vi "RT Loop - Acquisition and Logging.vi"(8 "error in (no error)":errorcluster, 9 "Acquisition and Logging Configuration":T1={"Data Rate"=1, "Samples per Read"=0, "Number of Reads to Save"=0, "Data File Name"="", "TDMS Properties"=[], "Number of Channels"=4, "Channel Scale Array"=[0.0, 0.0, 0.0, 0.0], "Channel Names"=[], "Trigger - RMS Value"=0.0, "Trigger - Channel"=0, "Trigger - Time (Minute)"=0} {"Data Rate" items=["51.200 kS/s (NI 9234)"=1, "25.600 kS/s (NI 9234)"=2, "17.067 kS/s (NI 9234)"=3, "12.800 kS/s (NI 9234)"=4, "10.240 kS/s (NI 9234)"=5, "8.533 kS/s (NI 9234)"=6, "7.314 kS/s (NI 9234)"=7, "6.400 kS/s (NI 9234)"=8, "5.689 kS/s (NI 9234)"=9, "5.120 kS/s (NI 9234)"=10, "4.654 kS/s (NI 9234)"=11, "4.267 kS/s (NI 9234)"=12, "3.938 kS/s (NI 9234)"=13, "3.657 kS/s (NI 9234)"=14, "3.413 kS/s (NI 9234)"=15, "3.200 kS/s (NI 9234)"=16, "3.012 kS/s (NI 9234)"=17, "2.845 kS/s (NI 9234)"=18, "2.695 kS/s (NI 9234)"=19, "2.560 kS/s (NI 9234)"=20, "2.438 kS/s (NI 9234)"=21, "2.328 kS/s (NI 9234)"=22, "2.226 kS/s (NI 9234)"=23, "2.133 kS/s (NI 9234)"=24, "2.048 kS/s (NI 9234)"=25, "1.969 kS/s (NI 9234)"=26, "1.896 kS/s (NI 9234)"=27, "1.829 kS/s (NI 9234)"=28, "1.765 kS/s (NI 9234)"=29, "1.707 kS/s (NI 9234)"=30, "1.652 kS/s (NI 9234)"=31]}, 10 "Acquisition and Logging Queue":refnum<queue>, 11 "Message Queue":refnum<queue>) -> ()   [LabVIEW 2020]
uses:
  support/Message Queue/Message Cluster.ctl
  controls/Acquisition and Logging Configuration.ctl
  <vilib>/LabVIEW Targets/FPGA/cRIO/shared/nicrio_ModuleControls/nicrio_cRIO-9234_DataRatesRing2.ctl
  controls/TDMS Properties.ctl
  controls/FPGA VI Reference.ctl
  Globals/Global - Configuration Options.vi
  Globals/Global - Monitoring Variables.vi
  <vilib>/rvi/errors/niLvFpgaAdjustHostInterfaceError.vi
  <vilib>/rvi/interface/nirviReadWriteControl/nirviReadWriteControl.xnode
  FPGA Bitfiles/forthexerciseemc_FPGATarget2_FPGAMain_d5JOh9LSVOQ.lvbitx
  support/Message Queue/Message Queue.lvlib
  NiFpgaLv.dll
panel:
  in  "Unbalanced Fan Speed 2":fxp<+/-,20,5>
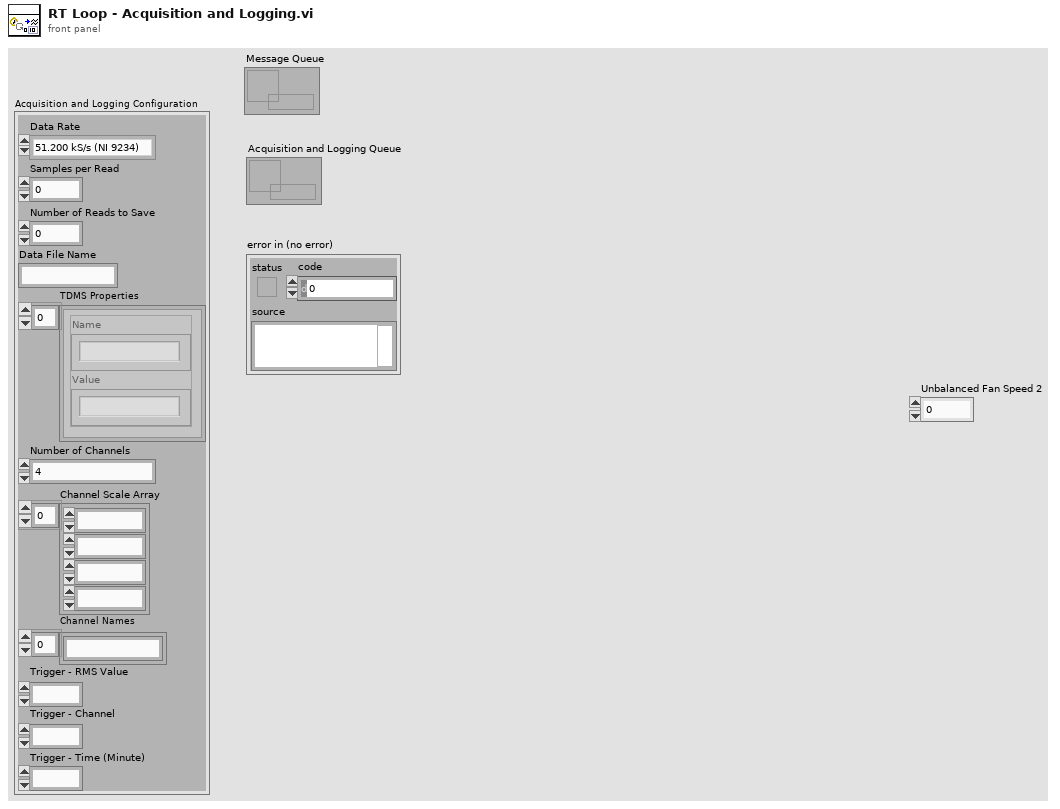
[diagram p1: front panel]
types:
  T1 = typedef "Acquisition and Logging Configuration.ctl" = cluster{"Data Rate":T2, "Samples per Read":i32, "Number of Reads to Save":i32, "Data File Name":string, "TDMS Properties":T3[], "Number of Channels":i32, "Channel Scale Array":fxp<+,24,12>[], "Channel Names":string[], "Trigger - RMS Value":dbl, "Trigger - Channel":i32, "Trigger - Time (Minute)":i32}
  T2 = typedef "nicrio_cRIO-9234_DataRatesRing2.ctl" = u8
  T3 = typedef "TDMS Properties.ctl" = cluster{"Name":string, "Value":string}
  T4 = typedef "FPGA VI Reference.ctl" = refnum<k20>
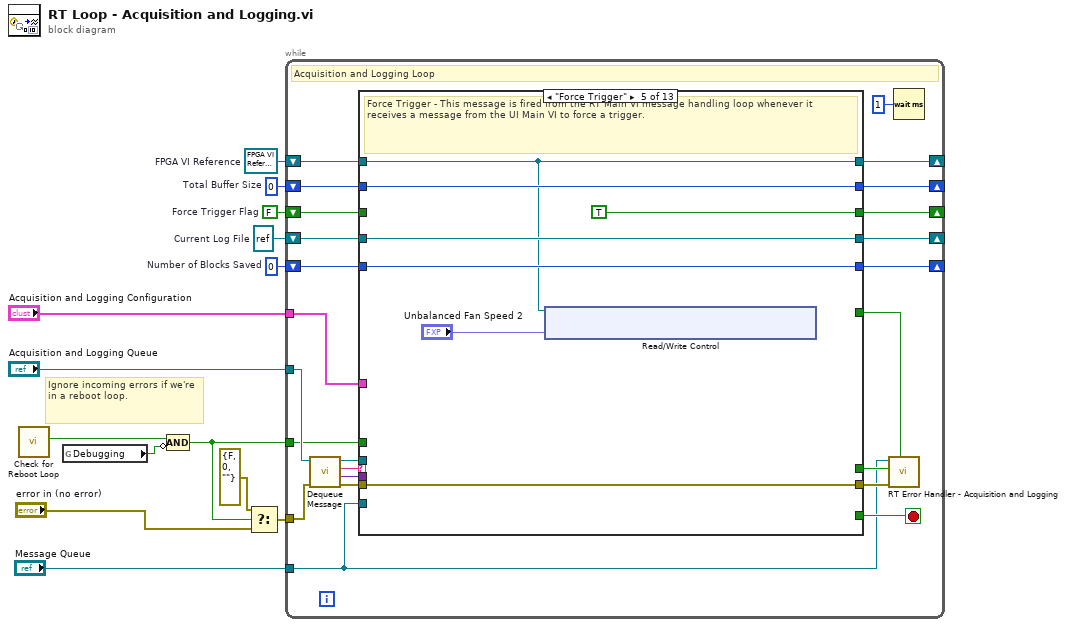
[diagram p0: block diagram]
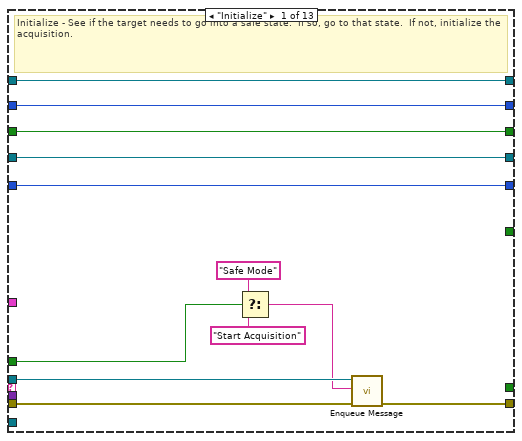
[diagram p2: hidden frame]
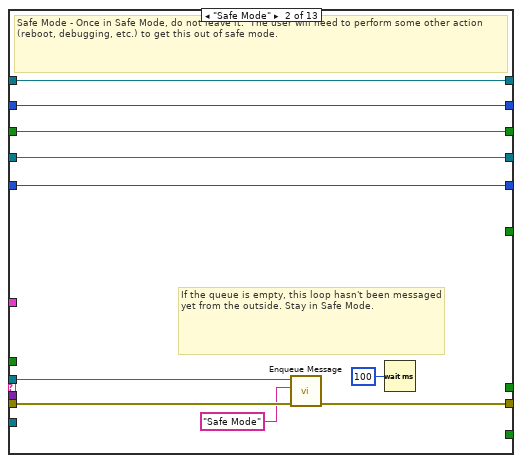
[diagram p3: hidden frame]
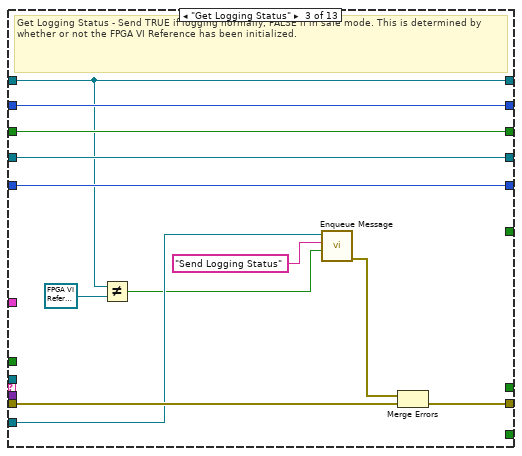
[diagram p4: hidden frame]
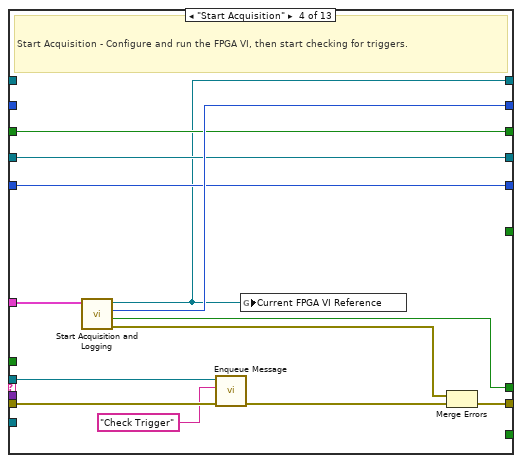
[diagram p5: hidden frame]
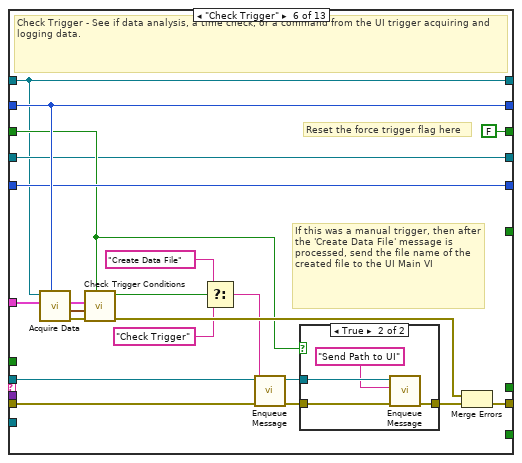
[diagram p6: hidden frame]
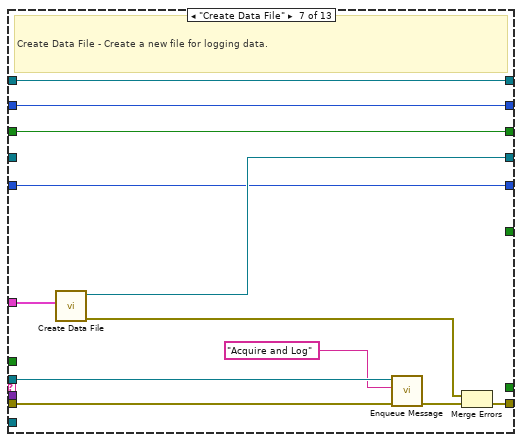
[diagram p8: hidden frame]
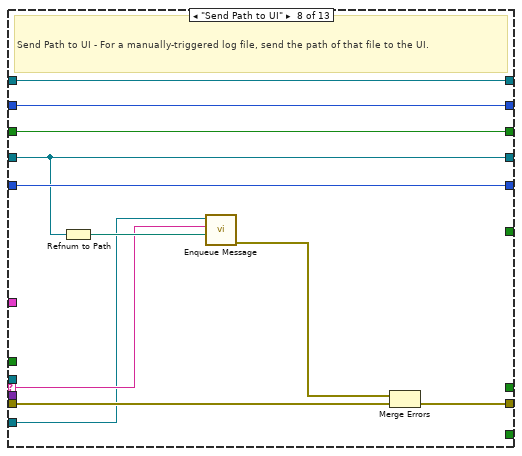
[diagram p9: hidden frame]
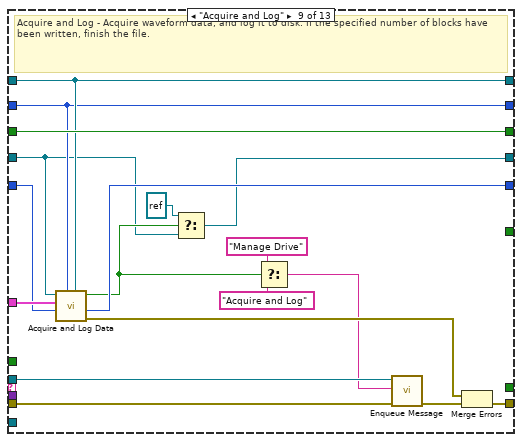
[diagram p10: hidden frame]
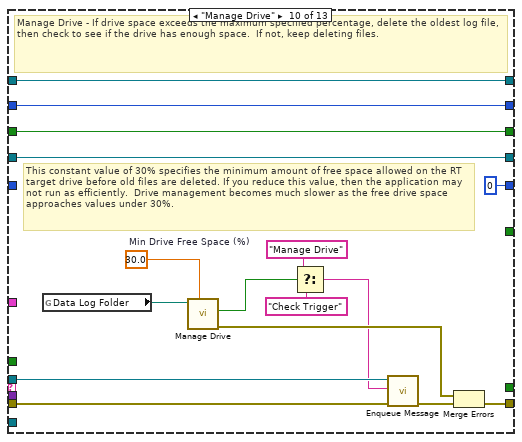
[diagram p11: hidden frame]
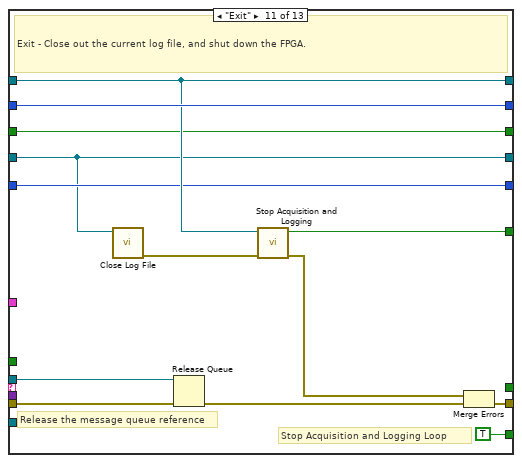
[diagram p12: hidden frame]
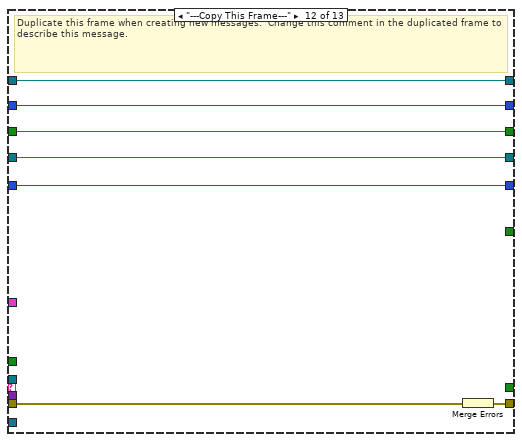
[diagram p13: hidden frame]
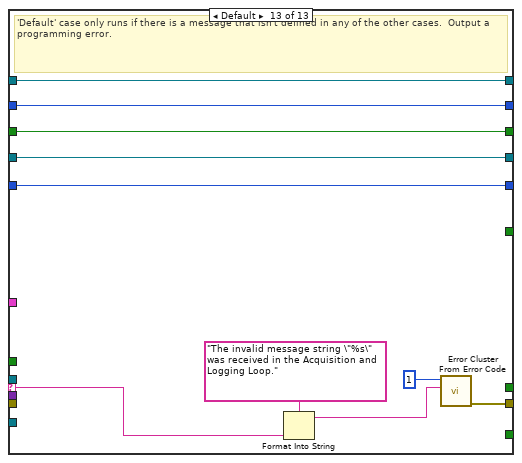
[diagram p14: hidden frame]
diagram:
  w7 = 0  # Number of Blocks Saved
  w8 = refnum<k34> refnum  # Current Log File
  w9 = FALSE  # Force Trigger Flag
  w11 = 0  # Total Buffer Size
  w12 = T4 refnum  # FPGA VI Reference
  # "Ignore incoming errors if we're in a reboot loop."
  n1 = call "Check for Reboot Loop.vi"() -> ("Start in Safe Mode?"=w3:bool)  [unwired: 10 in, 1 out]
  n2 = global read "Global - Configuration Options.vi" "Debugging"() -> (w2:bool)
  n3 = Compound Arithmetic op=AND(w3, invert w2) -> (w1:bool)
  n4 = Select(t=errorcluster {"status"=FALSE, "code"=0, "source"=""}, s=w1, f="error in (no error)") -> (s? t:f=w5:errorcluster)
  n5 = while {
    tunnel: "Acquisition and Logging Queue" -> [w34]
    tunnel: "Message Queue" -> [w18]
    shift-right: [w29] -> _
    shift-left: w12 -> [w31]
    shift-right: [w28] -> _
    shift-left: w11 -> [w30]
    tunnel: "Acquisition and Logging Configuration" -> [w27]
    shift-right: [w23] -> _
    shift-left: w9 -> [w24]
    shift-right: [w21] -> _
    shift-left: w8 -> [w22]
    shift-right: [w19] -> _
    shift-left: w7 -> [w20]
    tunnel: w5 -> [w16]
    tunnel: w1 -> [w15]
    stop <- w38 stop-if-true
    # "Acquisition and Logging Loop"
    n6 = call "Dequeue Message.vi"("error in (no error)"=w16, "Message Queue"=w34) -> ("error out"=w37:errorcluster, "Message Data"=w35:variant, "Message"=w36:string, "dup Message Queue"=w32:refnum<queue>)  [unwired: 6 in]
    n7 = case "Message Cases" shown="\"Force Trigger\"" w36 {
      selector: w36 -> [_ _ _ _ _ _ _ w134 _ _ _ _ w204]
      tunnel: w32 -> [w47 w57 _ w78 _ w105 w125 _ w156 w168 w188 _ _]
      tunnel: w37 -> [w48 w58 w72 w85 w92 w113 w129 w141 w159 w175 w184 w195 _]
      tunnel: [w40 w56 w64 w83 w92 w112 w128 w132 w158 w171 w185 w194 w202] -> w33
      tunnel: [_ _ _ _ _ _ _ _ _ _ TRUE _ _] -> w38
      tunnel: w35 -> [_ _ _ _ _ _ _ _ _ _ _ _ _]
      tunnel: w31 -> [w50 w60 w67 _ w86 w93 w130 w140 w149 w174 w182 w193 w200]
      tunnel: w30 -> [w49 w59 w71 _ w91 w110 w127 w139 w148 w173 w183 w192 w199]
      tunnel: [w50 w60 w67 w73 w86 w93 w130 w140 w149 w174 w182 w193 w200] -> w29
      tunnel: [w49 w59 w71 w80 w91 w110 w127 w139 w148 w173 w183 w192 w199] -> w28
      tunnel: w27 -> [_ _ _ w84 _ w111 w122 _ w154 _ _ _ _]
      tunnel: [_ _ _ w81 _ _ _ _ _ _ _ _ _] -> w25
      tunnel: w24 -> [w43 w55 w70 w76 _ w95 w123 w138 w155 w161 w180 w191 w198]
      tunnel: [w43 w55 w70 w76 TRUE ("Force Trigger Flag") FALSE ("Force Trigger Flag") w123 w138 w155 w161 w180 w191 w198] -> w23
      tunnel: w22 -> [w42 w54 w69 w75 w90 w94 _ w136 w144 w172 w177 w190 w197]
      tunnel: [w42 w54 w69 w75 w90 w94 w120 w136 w143 w172 w177 w190 w197] -> w21
      tunnel: w20 -> [w41 w53 w68 w74 w88 w100 w119 w137 w147 _ w179 w189 w196]
      tunnel: [w41 w53 w68 w74 w88 w100 w119 w137 w146 0 ("Number of Blocks Saved") w179 w189 w196] -> w19
      tunnel: w18 -> [_ _ w65 _ _ _ _ w133 _ _ _ _ _]
      tunnel: [_ _ _ _ _ _ _ _ _ _ w176 _ _] -> w17
      tunnel: w15 -> [w39 _ _ _ _ _ _ _ _ _ _ _ _]
      frame "Initialize" {
        # "Initialize - See if the target needs to go into a safe state.  If so, go to that state.  If not, initialize the acquisition."
        n8 = Select(t="Safe Mode", s=w39, f="Start Acquisition") -> (s? t:f=w44:string)
        n9 = call "Enqueue Message.vi"("error in (no error)"=w48, "Message"=w44, "Message Queue"=w47) -> ("error out"=w40:errorcluster)  [unwired: 7 in, 1 out]
      }
      frame "Safe Mode" {
        # "If the queue is empty, this loop hasn't been messaged yet from the outside. Stay in Safe Mode."
        # "Safe Mode - Once in Safe Mode, do not leave it.  The user will need to perform some other action (reboot, debugging, etc.) to get this out of safe mode."
        n10 = call "Enqueue Message.vi"("error in (no error)"=w58, "Message"="Safe Mode", "Message Queue"=w57) -> ("error out"=w56:errorcluster)  [unwired: 7 in, 1 out]
        n11 = Wait (ms)(milliseconds to wait=u32 100) -> ()  [unwired: 1 out]
      }
      frame "Get Logging Status" {
        # "Get Logging Status - Send TRUE if logging normally, FALSE if in safe mode. This is determined by whether or not the FPGA VI Reference has been initialized."
        n12 = Not Equal?(x=w67, y=T4 refnum ("FPGA VI Reference")) -> (x != y?=w62:bool)
        n13 = call "Enqueue Message.vi"("Message Data"=w62, "Message"="Send Logging Status", "Message Queue"=w65) -> ("error out"=w63:errorcluster)  [unwired: 7 in, 1 out]
        n14 = Merge Errors(w63, w72) -> (w64:errorcluster)
      }
      frame "Start Acquisition" {
        # "Start Acquisition - Configure and run the FPGA VI, then start checking for triggers."
        n15 = call "Start Acquisition and Logging.vi"("Acquisition and Logging Configuration"=w84) -> ("error out"=w82:errorcluster, "Wait on IRQ Timeout?"=w81:bool, "Total Buffer Size"=w80:i32, "FPGA VI Reference Out"=w73:T4)  [unwired: 7 in]
        n16 = call "Enqueue Message.vi"("error in (no error)"=w85, "Message"="Check Trigger", "Message Queue"=w78) -> ("error out"=w79:errorcluster)  [unwired: 7 in, 1 out]
        n17 = global write "Global - Monitoring Variables.vi" "Current FPGA VI Reference"(w73) -> ()
        n18 = Merge Errors(w82, w79) -> (w83:errorcluster)
      }
      frame "Force Trigger" {
        # "Force Trigger - This message is fired from the RT Main VI message handling loop whenever it receives a message from the UI Main VI to force a trigger."
        n19 = xnode "Read/Write Control"("FPGA VI Reference In"=w86, "Unbalanced Fan Speed"="Unbalanced Fan Speed 2") -> ()  [unwired: 1 in, 2 out]
      }
      frame "Check Trigger" {
        # "If this was a manual trigger, then after the 'Create Data File' message is processed, send the file name of the created file to the UI Main VI"
        # "Reset the force trigger flag here"
        # "Check Trigger - See if data analysis, a time check, or a command from the UI trigger acquiring and logging data."
        n20 = call "Acquire Data.vi"("Total Buffer Size"=w110, "Acquisition and Logging Configuration"=w111, "FPGA VI Reference"=w93) -> ("error out"=w108:errorcluster, "Waveform Data"=w107:waveform(sgl)[], "dup Acquisition and Logging Configuration"=w106:T1)  [unwired: 6 in]
        n21 = call "Check Trigger Conditions.vi"("Force Trigger?"=w95, "error in (no error)"=w108, "Waveform Data"=w107, "Acquisition and Logging Configuration"=w106) -> ("error out"=w109:errorcluster, "Trigger Condition Met?"=w104:bool)  [unwired: 6 in]
        n22 = Select(t="Create Data File", s=w104, f="Check Trigger") -> (s? t:f=w101:string)
        n23 = call "Enqueue Message.vi"("error in (no error)"=w113, "Message"=w101, "Message Queue"=w105) -> ("error out"=w98:errorcluster, "dup Message Queue"=w96:refnum<queue>)  [unwired: 7 in]
        n24 = case shown="True" w95 {
          tunnel: w98 -> [w114 w117]
          tunnel: [w114 w118] -> w97
          tunnel: w96 -> [_ w116]
          frame False {
          }
          frame True {
            n25 = call "Enqueue Message.vi"("error in (no error)"=w117, "Message"="Send Path to UI", "Message Queue"=w116) -> ("error out"=w118:errorcluster)  [unwired: 7 in, 1 out]
          }
        }
        n26 = Merge Errors(w109, w97) -> (w112:errorcluster)
      }
      frame "Create Data File" {
        # "Create Data File - Create a new file for logging data."
        n27 = call "Create Data File.vi"("Acquisition and Logging Configuration"=w122) -> ("error out"=w121:errorcluster, "TDMS File Reference"=w120:refnum<k34>)  [unwired: 9 in]
        n28 = call "Enqueue Message.vi"("error in (no error)"=w129, "Message"="Acquire and Log", "Message Queue"=w125) -> ("error out"=w126:errorcluster)  [unwired: 7 in, 1 out]
        n29 = Merge Errors(w121, w126) -> (w128:errorcluster)
      }
      frame "Send Path to UI" {
        # "Send Path to UI - For a manually-triggered log file, send the path of that file to the UI."
        n30 = Refnum to Path(1:w136) -> (0:w135:path)
        n31 = call "Enqueue Message.vi"("Message Data"=w135, "Message"=w134, "Message Queue"=w133) -> ("error out"=w131:errorcluster)  [unwired: 7 in, 1 out]
        n32 = Merge Errors(w131, w141) -> (w132:errorcluster)
      }
      frame "Acquire and Log" {
        # "Acquire and Log - Acquire waveform data, and log it to disk. If the specified number of blocks have been written, finish the file."
        n33 = call "Acquire and Log Data.vi"("FPGA VI Reference"=w149, "Total Buffer Size"=w148, "Number of Blocks Saved in"=w147, "Acquisition and Logging Configuration"=w154, "TDMS File Reference"=w144) -> ("error out"=w153:errorcluster, "Number of Blocks Saved out"=w146:i32, "Logging Complete?"=w145:bool)  [unwired: 4 in]
        n34 = Select(t=refnum<k34> refnum, s=w145, f=w144) -> (s? t:f=w143:refnum<k34>)
        n35 = Select(t="Manage Drive", s=w145, f="Acquire and Log") -> (s? t:f=w150:string)
        n36 = call "Enqueue Message.vi"("error in (no error)"=w159, "Message"=w150, "Message Queue"=w156) -> ("error out"=w157:errorcluster)  [unwired: 7 in, 1 out]
        n37 = Merge Errors(w153, w157) -> (w158:errorcluster)
      }
      frame "Manage Drive" {
        w170 = 30.0  # Min Drive Free Space (%)
        # "This constant value of 30% specifies the minimum amount of free space allowed on the RT target drive before old files are deleted. If you reduce this value, then the application may not run as efficiently.  Drive management becomes much slower as the free drive space approaches values under 30%."
        # "Manage Drive - If drive space exceeds the maximum specified percentage, delete the oldest log file, then check to see if the drive has enough space.  If not, keep deleting files."
        n38 = global read "Global - Configuration Options.vi" "Data Log Folder"() -> (w160:path)
        n39 = call "Manage Drive.vi"("Min Drive Free Space (%)"=w170, "Data Folder"=w160) -> ("error out"=w167:errorcluster, "Drive Space Below Limit"=w166:bool)  [unwired: 8 in]
        n40 = Select(t="Manage Drive", s=w166, f="Check Trigger") -> (s? t:f=w163:string)
        n41 = call "Enqueue Message.vi"("error in (no error)"=w175, "Message"=w163, "Message Queue"=w168) -> ("error out"=w169:errorcluster)  [unwired: 7 in, 1 out]
        n42 = Merge Errors(w167, w169) -> (w171:errorcluster)
      }
      frame "Exit" {
        # "Stop Acquisition and Logging Loop"
        # "Release the message queue reference"
        # "Exit - Close out the current log file, and shut down the FPGA."
        n43 = call "Close Log File.vi"("Log File"=w177) -> ("error out"=w178:errorcluster)  [unwired: 10 in]
        n44 = Release Queue(queue=w188, error in (no error)=w184) -> (error out=w186:errorcluster)  [unwired: 1 in, 2 out]
        n45 = call "Stop Acquisition and Logging.vi"("error in (no error)"=w178, "FPGA VI Reference"=w182) -> ("error out"=w181:errorcluster, "Stop FPGA Timeout?"=w176:bool)  [unwired: 8 in]
        n46 = Merge Errors(w181, w186) -> (w185:errorcluster)
      }
      frame "---Copy This Frame---" {
        # "Duplicate this frame when creating new messages.  Change this comment in the duplicated frame to describe this message."
        n47 = Merge Errors(w195) -> (w194:errorcluster)
      }
      frame Default {
        # "'Default' case only runs if there is a message that isn't defined in any of the other cases.  Output a programming error."
        n48 = Format Into String(format string="The invalid message string \"%s\" was received in the Acquisition and Logging Loop." ("Unknown Message Error Text"), w204) -> (resulting string=w201:string)  [unwired: 2 in, 1 out]
        n49 = call <vilib>:"Error Cluster From Error Code.vi"("error message (\"\")"=w201, "error code (0)"=1) -> ("error out"=w202:errorcluster)  [unwired: 7 in]
      }
    }
    n50 = call "RT Error Handler - Acquisition and Logging.vi"("Stop FPGA Timeout"=w17, "error in (no error)"=w33, "IRQ Timeout"=w25, "Message Queue"=w18) -> ()  [unwired: 7 in, 1 out]
    n51 = Wait (ms)(milliseconds to wait=u32 1) -> ()  [unwired: 1 out]
  }
